vi "串口.vi"(5 "byte count":u32, 7 "case":T1(ring)=enum."change", 8 "error in":errorcluster, 9 "baud rate (9600)":u32=115200 caption="波特率(115200)", 10 "write buffer":string, 11 "VISA name":refnum<visa-resource-name>) -> (0 "error out":errorcluster, 1 "empty?":bool, 2 "read buffer":string, 3 "VISA resource name out":refnum<visa-resource-name>)   [LabVIEW 2016]
uses:
  <vilib>/Instr/_visa.llb/VISA Configure Serial Port (Instr).vi
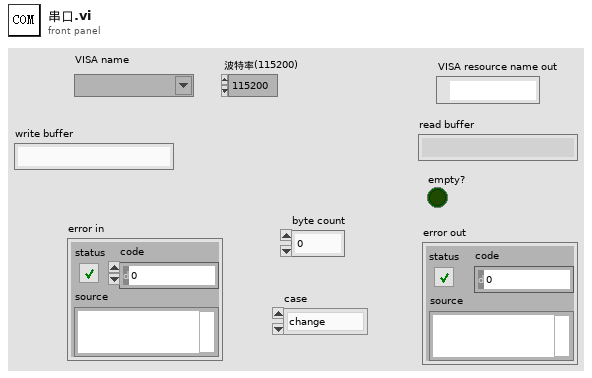
[diagram p1: front panel]
types:
  T1 = enum16{"initial", "write", "read", "release", "change"}
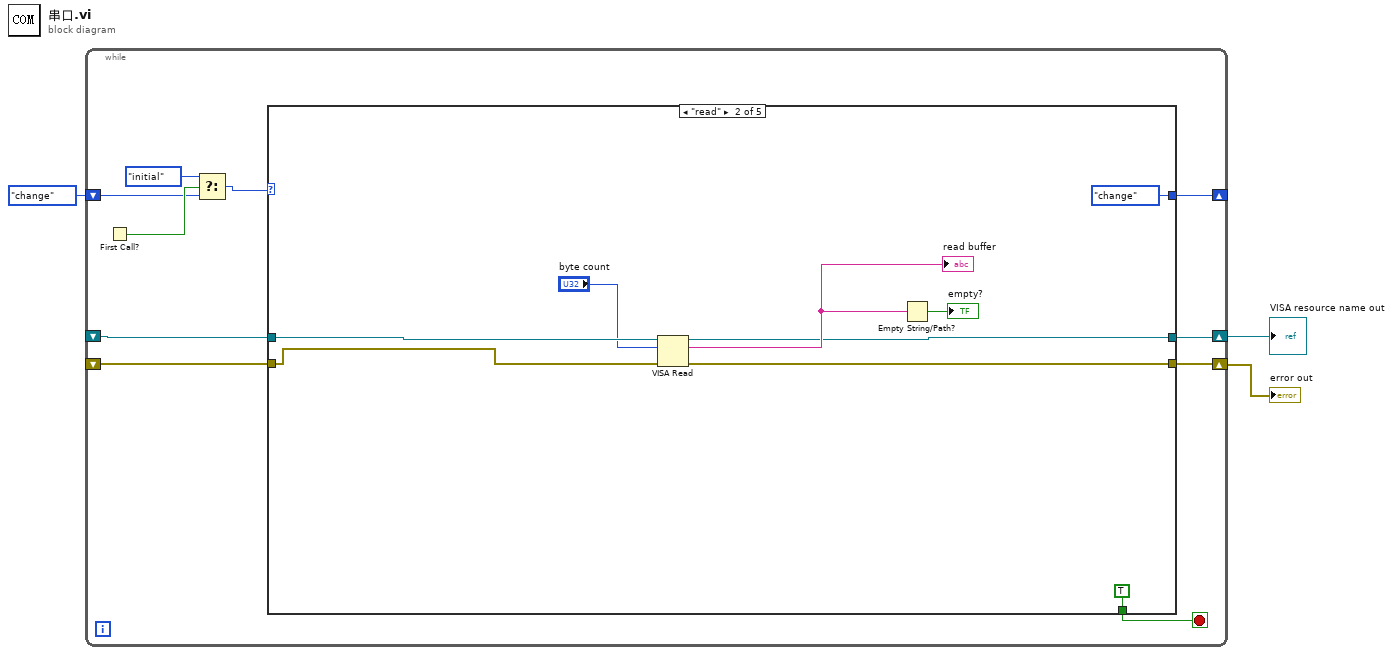
[diagram p0: block diagram]
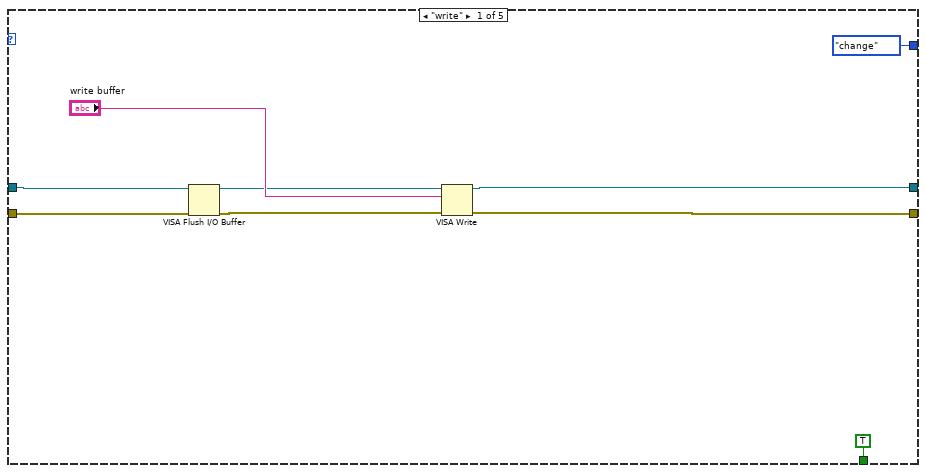
[diagram p2: hidden frame]
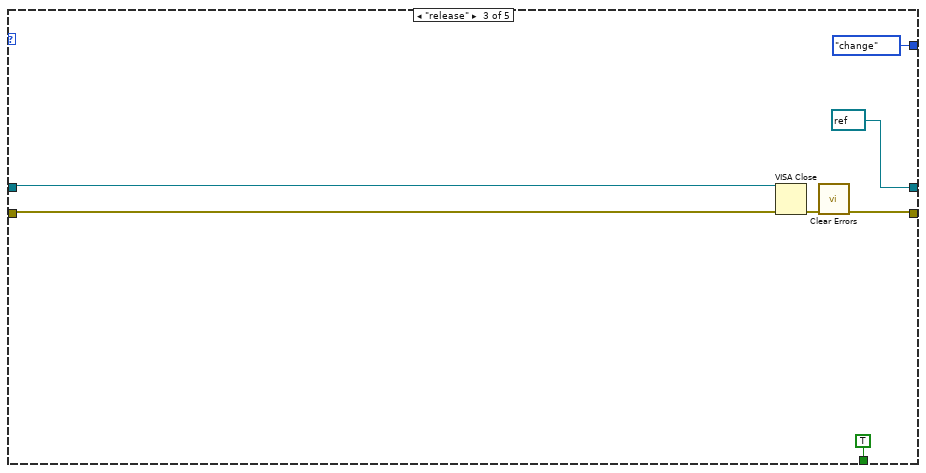
[diagram p3: hidden frame]
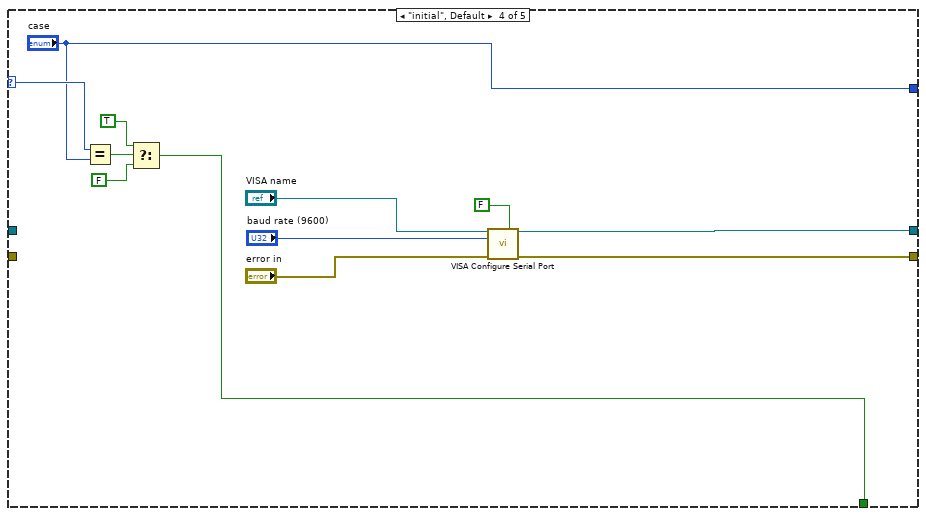
[diagram p4: hidden frame]
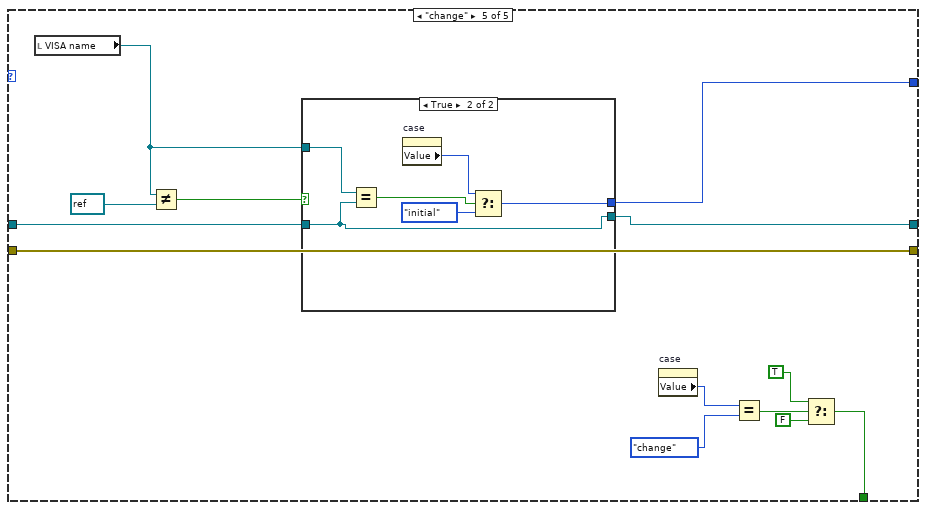
[diagram p5: hidden frame]
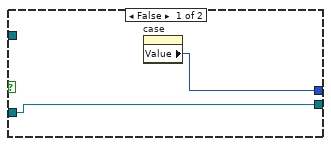
[diagram p6: hidden frame]
diagram:
  n1 = while {
    shift-right: [w12] -> w1
    shift-left: _ -> [w11]
    shift-right: [w10] -> w3
    shift-left: _ -> [w9]
    shift-right: [w6] -> _
    shift-left: T1."change" ("f") -> [w7]
    stop <- w4 stop-if-true
    n2 = First Call?() -> (First Call?: T/F=w13:bool)
    n3 = Select(t=T1."initial", s=w13, f=w7) -> (s? t:f=w8:T1)
    n4 = case shown="\"read\"" w8 {
      selector: w8 -> [_ _ _ w42 _]
      tunnel: [w18 w27 refnum<visa-resource-name> refnum ("VISA resource name out") w45 w51] -> w12
      tunnel: w11 -> [w21 w23 w32 _ w52]
      tunnel: w9 -> [w20 w24 w37 _ w61]
      tunnel: [w19 w28 w36 w44 w61] -> w10
      tunnel: [T1."change" ("f") T1."change" ("f") T1."change" ("f") "case" w62] -> w6
      tunnel: [TRUE ("f") TRUE ("f") TRUE w38 w55] -> w4
      frame "write" {
        n5 = VISA Flush I/O Buffer(VISA resource name=w21) -> (VISA resource name out=w14:refnum<visa-resource-name>)  [unwired: 2 in, 1 out]
        n6 = VISA Write(VISA resource name=w14, write buffer="write buffer", error in (no error)=w20) -> (VISA resource name out=w18:refnum<visa-resource-name>, error out=w19:errorcluster)  [unwired: 1 out]
      }
      frame "read" {
        n7 = VISA Read(VISA resource name=w23, byte count="byte count", error in (no error)=w24) -> (VISA resource name out=w27:refnum<visa-resource-name>, read buffer=w29:string, error out=w28:errorcluster)  [unwired: 1 out]
        "read buffer" <- w29
        n8 = Empty String/Path?(string/path=w29) -> (empty?=→"empty?":bool)
      }
      frame "release" {
        n9 = VISA Close(VISA resource name=w32, error in (no error)=w37) -> (error out=w31:errorcluster)
        n10 = call <vilib>:"Clear Errors.vi"("error in (no error)"=w31) -> ("error out"=w36:errorcluster)  [unwired: 5 in, 1 out]
      }
      frame "initial", Default {
        n11 = Equal?(x=w42, y="case") -> (x = y?=w43:bool)
        n12 = Select(t=TRUE, s=w43, f=FALSE) -> (s? t:f=w38:bool)
        n13 = call-poly "VISA Configure Serial Port"("VISA resource name"="VISA name", "Enable Termination\nChar (T)"=FALSE ("Enable Termination\nChar (T)"), "baud rate (9600)"="baud rate (9600)", "error in (no error)"="error in") -> ("VISA resource name out"=w45:refnum<visa-resource-name>, "error out"=w44:errorcluster)  [unwired: 10 in]
      }
      frame "change" {
        n14 = local read "VISA name"() -> (w50:refnum<visa-resource-name>)
        n15 = Not Equal?(x=w50, y=refnum<visa-resource-name> refnum) -> (x != y?=w54:bool)
        n16 = case shown="True" w54 {
          tunnel: [w63 w67] -> w62
          tunnel: w52 -> [w64 w65]
          tunnel: [w64 w65] -> w51
          tunnel: w50 -> [_ w66]
          frame False {
            n17 = property on="case" class="Enum (strict)"() -> ("Value"=w63:T1)  [unwired: 2 in, 2 out]
          }
          frame True {
            n18 = Equal?(x=w66, y=w65) -> (x = y?=w68:bool)
            n19 = property on="case" class="Enum (strict)"() -> ("Value"=w70:T1)  [unwired: 2 in, 2 out]
            n20 = Select(t=w70, s=w68, f=T1."initial") -> (s? t:f=w67:T1)
          }
        }
        n21 = property on="case" class="Enum (strict)"() -> ("Value"=w60:T1)  [unwired: 2 in, 2 out]
        n22 = Equal?(x=w60, y=T1."change") -> (x = y?=w58:bool)
        n23 = Select(t=TRUE, s=w58, f=FALSE) -> (s? t:f=w55:bool)
      }
    }
  }
  "error out" <- w3
  "VISA resource name out" <- w1
